vi "StopAcquisition.vi"(8 "error in (no error)":errorcluster, 11 "NIScope in":refnum<class "NIScope.lvclass">) -> (0 "error out":errorcluster, 3 "NIScope out":refnum<class "NIScope.lvclass">)   [LabVIEW 2018, in "ScopePlugins.lvlib" / "NIScope.lvclass"]
doc: "Stops the acquisition of measurements from the instrument."
uses:
  NIScope.lvclass
  C:/Users/ico/Documents/Projects/NistPluggableModules/Scope/ScopePlugins/ScopePluginBaseClass/ScopePluginsBase.lvclass
  ScopePluginBaseClass/ScopePluginsBase.lvclass/ScopePluginsBase.ctl
  ScopePluginBaseClass/Accessors/Write Channels.vi
  ScopePluginBaseClass/Accessors/Read Channels.vi
  ScopePluginBaseClass/ScopePluginsBase.lvclass
  <instrlib>/niSync/niSync.llb/niSync Read Trigger Time Stamp (Single).vi
panel:
  out "time stamp out":timestamp
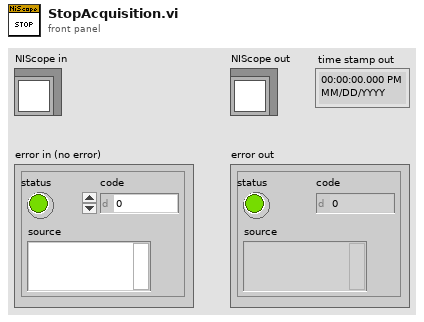
[diagram p1: front panel]
types:
  T1 = typedef "ScopePlugins.lvlib/ScopePluginsBase.lvclass/ChannelSetting(s).ctl" = cluster{"Number of Channels":i32, "Channel(s)":cluster{"Enabled":bool, "Instrument Handle":string, "Channel Name":string, "Maximum Input Frequency":dbl, "Verticle Settings":cluster{"Vertical Range":dbl, "Vertical Offset":dbl, "Probe Attenuation":dbl, "Vertical Coupling":i32}, "Connected":bool, "Input Impedance":dbl, "IO Type Instrument Handle":refnum<k15>}[]}
  T2 = cluster{"Enabled":bool, "Instrument Handle":string, "Channel Name":string, "Maximum Input Frequency":dbl, "Verticle Settings":cluster{"Vertical Range":dbl, "Vertical Offset":dbl, "Probe Attenuation":dbl, "Vertical Coupling":i32}, "Connected":bool, "Input Impedance":dbl, "IO Type Instrument Handle":refnum<k15>}[]
  T3 = cluster{"Enabled":bool, "Instrument Handle":string, "Channel Name":string, "Maximum Input Frequency":dbl, "Verticle Settings":cluster{"Vertical Range":dbl, "Vertical Offset":dbl, "Probe Attenuation":dbl, "Vertical Coupling":i32}, "Connected":bool, "Input Impedance":dbl, "IO Type Instrument Handle":refnum<k15>}
  T4 = typedef "ScopePlugins.lvlib/ScopePluginsBase.lvclass/Sync.ctl" = cluster{"Handle":string, "SrcTerm":string, "DestTerm":string}
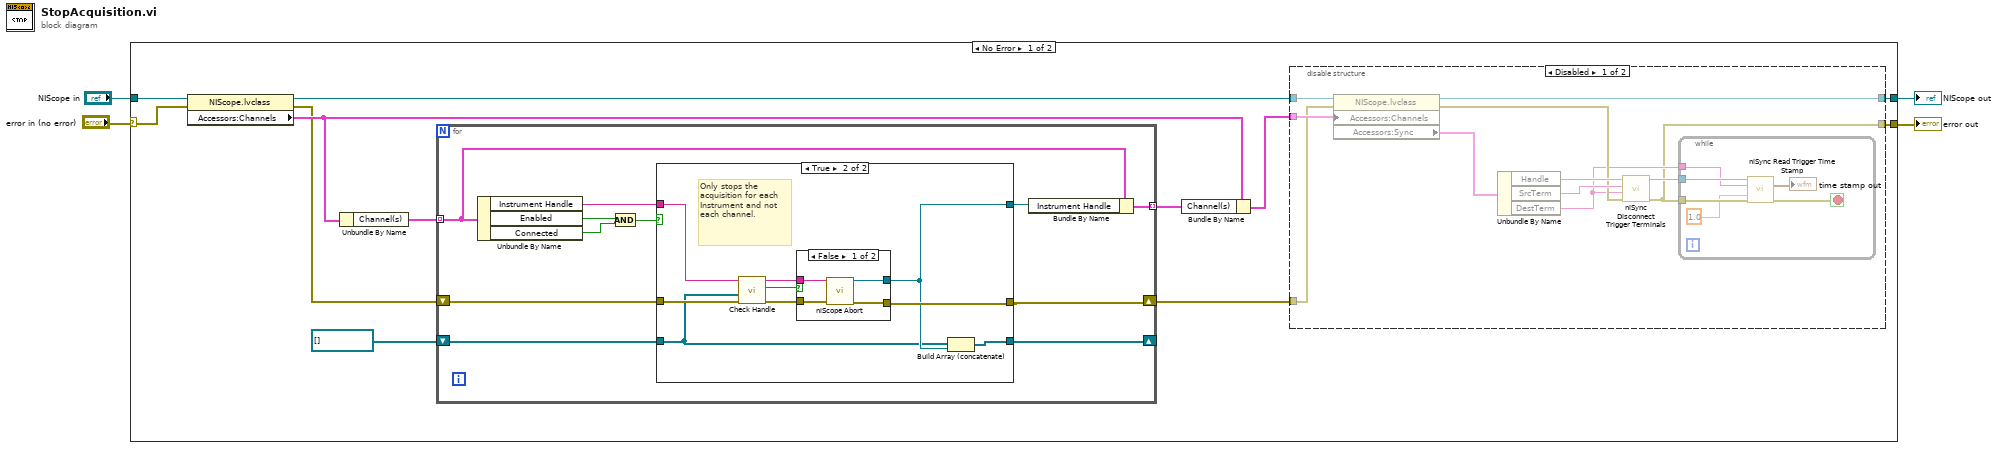
[diagram p0: block diagram]
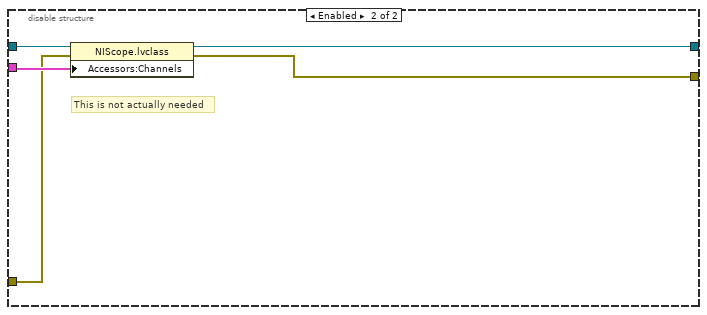
[diagram p4: hidden frame]
diagram:
  n1 = case shown="No Error" "error in (no error)" {
    selector: "error in (no error)" -> [w14 w68]
    tunnel: "NIScope in" -> [w16 w69]
    tunnel: [w6 w68] -> w2
    tunnel: [w12 w69] -> w1
    frame No Error {
      n2 = property class="NIScope.lvclass"(reference=w16, error in=w14) -> (reference out=w15:refnum<class "NIScope.lvclass">, error out=w8:errorcluster, "Accessors:Channels"=w10:T1)
      n3 = Unbundle By Name(w10) -> ("Channel(s)"=w9:T2)
      n4 = for {
        shift-right: [w23] -> w5
        shift-left: w8 -> [w26]
        tunnel: w9 -> [w27] mode=indexing
        shift-right: [w24] -> _
        shift-left: refnum<k15>[] [] -> [w25]
        tunnel: [w20] -> w7 mode=indexing
        n5 = Unbundle By Name(w27) -> ("Instrument Handle"=w22:string, "Enabled"=w19:bool, "Connected"=w18:bool)
        n6 = And(x=w19, y=w18) -> (x .and. y?=w17:bool)
        n7 = case shown="True" w17 {
          tunnel: w22 -> [w30 w33]
          tunnel: w25 -> [w29 w34]
          tunnel: [w29 w39] -> w24
          tunnel: w26 -> [w28 w36]
          tunnel: [w28 w38] -> w23
          tunnel: [w30 w37] -> w21
          frame False {
          }
          frame True {
            # "Only stops the \nacquisition for each\nInstrument and not\neach channel."
            n8 = call "Check Handle.vi"("error in (no error)"=w36, "Array"=w34, "Handle In"=w33) -> ("error out"=w35:errorcluster, "Duplicate Instrument?"=w32:bool, "Handle Out"=w31:string)  [unwired: 6 in]
            n9 = case shown="False" w32 {
              tunnel: w35 -> [w43 w45]
              tunnel: [w42 w45] -> w38
              tunnel: [w41 w44] -> w37
              tunnel: w31 -> [w40 w44]
              frame False {
                n10 = call <instrlib>:"niScope Abort.vi"("instrument handle"=w40, "error in"=w43) -> ("instrument handle out"=w41:refnum<k15>, "error out"=w42:errorcluster)  [unwired: 12 in]
              }
              frame True {
              }
            }
            n11 = Build Array (concatenate)(w34, w37) -> (w39:refnum<k15>[])
          }
        }
        n12 = Bundle By Name(cluster=w27, "Instrument Handle"=w21) -> (w20:T3)
      }
      n13 = Bundle By Name(cluster=w10, "Channel(s)"=w7) -> (w11:T1)
      n14 = disable-structure shown="Disabled" {
        disable-tunnel: w15 -> [w56 w67]
        disable-tunnel: [w55 w65] -> w12
        disable-tunnel: w11 -> [w54 w66]
        disable-tunnel: [w47 w63] -> w6
        disable-tunnel: w5 -> [w46 w64]
        frame Disabled {
          n15 = property class="NIScope.lvclass"(reference=w56, error in=w46, "Accessors:Channels"=w54) -> (reference out=w55:refnum<class "NIScope.lvclass">, error out=w50:errorcluster, "Accessors:Sync"=w53:T4)
          n16 = Unbundle By Name(w53) -> ("Handle"=w52:string, "SrcTerm"=w51:string, "DestTerm"=w48:string)
          n17 = call <instrlib>:"niSync Disconnect Trigger Terminals.vi"("error in (no error)"=w50, "destination terminal"=w48, "source terminal"=w51, "instrument handle"=w52) -> ("error out"=w47:errorcluster, "instrument handle out"=w49:refnum<k15>)  [unwired: 6 in]
          n18 = while {
            tunnel: w47 -> [w62]
            tunnel: w49 -> [w61]
            tunnel: w48 -> [w60]
            stop <- w58 stop-if-true
            n19 = call-poly <instrlib>:"niSync Read Trigger Time Stamp.vi"("instrument handle"=w61, "terminal"=w60, "timeout"=1.0, "error in (no error)"=w62) -> ("time stamp out"=→"time stamp out":timestamp, "error out"=w58:errorcluster)  [unwired: 8 in, 2 out]
          }
        }
        frame Enabled {
          # "This is not actually needed"
          n20 = property class="NIScope.lvclass"(reference=w67, error in=w64, "Accessors:Channels"=w66) -> (reference out=w65:refnum<class "NIScope.lvclass">, error out=w63:errorcluster)
        }
      }
    }
    frame Error {
    }
  }
  "error out" <- w2
  "NIScope out" <- w1
